vi "Validate Choice.vi"(8 "error in (no error)":errorcluster, 10 "Choice":T1, 11 "Reversi in":refnum<class "Reversi.lvclass">) -> (0 "error out":errorcluster, 3 "Reversi out":refnum<class "Reversi.lvclass">)   [LabVIEW 2020, in "Reversi.lvlib" / "Reversi.lvclass"]
uses:
  Reversi.lvclass
  Space Cluster.ctl
  Space Coordinates.ctl
  Space Ring.ctl
  Reversi.lvclass/Reversi.ctl
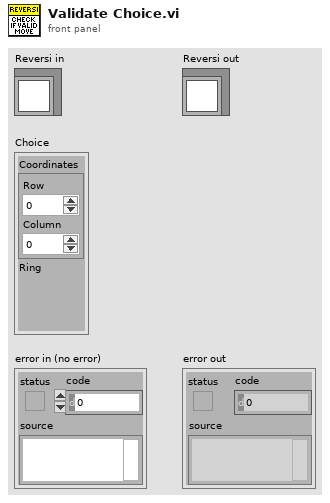
[diagram p1: front panel]
types:
  T1 = typedef "Reversi.lvlib/Reversi.lvclass/Space Cluster.ctl" = cluster{"Coordinates":T2, "Ring":T3}
  T2 = typedef "Reversi.lvlib/Reversi.lvclass/Space Coordinates.ctl" = cluster{"Row":i32, "Column":i32}
  T3 = typedef "Reversi.lvlib/Reversi.lvclass/Space Ring.ctl" = u16
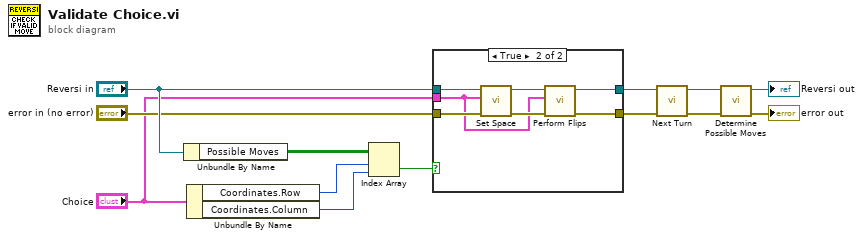
[diagram p0: block diagram]
diagram:
  n1 = Unbundle By Name("Reversi in") -> ("Possible Moves"=w12:bool[][])
  n2 = Unbundle By Name("Choice") -> ("Coordinates.Row"=w11:i32, "Coordinates.Column"=w10:i32)
  n3 = Index Array(array=w12, index (row)=w11, index (col)=w10) -> (element=w9:bool)
  n4 = case shown="True" w9 {
    tunnel: [w15 w17] -> w1
    tunnel: "Reversi in" -> [w15 w22]
    tunnel: "error in (no error)" -> [w14 w21]
    tunnel: [w14 w16] -> w2
    tunnel: "Choice" -> [_ w18]
    frame False {
    }
    frame True {
      n5 = call "Set Space.vi"("error in (no error)"=w21, "Space"=w18, "Reversi in"=w22) -> ("error out"=w19:errorcluster, "Reversi out"=w20:refnum<class "Reversi.lvclass">)  [unwired: 7 in]
      n6 = call "Perform Flips.vi"("error in (no error)"=w19, "Choice"=w18, "Reversi in"=w20) -> ("error out"=w16:errorcluster, "Reversi out"=w17:refnum<class "Reversi.lvclass">)  [unwired: 7 in]
    }
  }
  n7 = call "Next Turn.vi"("error in (no error)"=w2, "Reversi in"=w1) -> ("error out"=w5:errorcluster, "Reversi out"=w6:refnum<class "Reversi.lvclass">)  [unwired: 8 in]
  n8 = call "Determine Possible Moves.vi"("error in (no error)"=w5, "Reversi in"=w6) -> ("error out"=→"error out":errorcluster, "Reversi out"=→"Reversi out":refnum<class "Reversi.lvclass">)  [unwired: 8 in]
